vi "poly_cast_array_variant_U8.vi"(2 "array variant":variant[](array[variant])) -> (7 "data (255)":u8[](array[numeric]))   [LabVIEW 2015]
doc: "This vi attempts to cast a variant to data. The data is set to default value if an error occurs. This vi is intended to be used as a convenience tool when the data type is unambigous.\n\nWritten by Marcin Konowalczyk\nTimmel Group @ Oxford University"
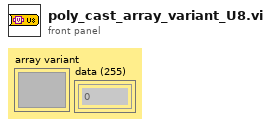
[diagram p1: front panel]
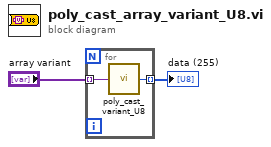
[diagram p0: block diagram]
diagram:
  n1 = for {
    tunnel: "array variant" -> [w4] mode=indexing
    tunnel: [w3] -> w1 mode=indexing
    n2 = call "poly_cast_variant_U8.vi"("variant"=w4) -> ("data (255)"=w3:u8)  [unwired: 8 in]
  }
  "data (255)" <- w1
